vi "RightDrive.vi"(10 "Effort":dbl=-0.007874015748031496) -> ()   [LabVIEW 2018]
uses:
  <vilib>/Rock Robotics/WPI/ThirdParty/Phoenix-LabVIEW/Motor Controller/Controls/CTRE_Phoenix_MotorControl_ControlMode.ctl
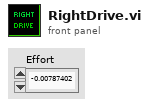
[diagram p1: front panel]
types:
  T1 = typedef "CTRE_Phoenix_MotorControl_ControlMode.ctl" = u16
  T2 = typedef "WPI_MotorControlDeviceRef.ctl" = cluster{"DeviceStatus":errorcluster, "Type":T3, "PWM":cluster{"PWM Channel":T4, "DeadBand":T5}, "CAN":cluster{"Device Number":u8, "SetOutput VI Ref":variant, "GetOutput VI Ref":variant, "Enable VI Ref":variant, "Disable VI Ref":variant, "Data":variant}, "Invert":bool, "DIO PWM":cluster{"PWM \"Enable\" Channel":T4, "DIOChannel":T6, "PWM Rate":dbl}}
  T3 = typedef "WPI_MotorControlType.ctl" = enum16{"PWM", "CAN", "DIO PWM"}
  T4 = typedef "FPGA_DIOPWMChannel.ctl" = enum8{"PWM 0", "PWM 1", "PWM 2", "PWM 3", "PWM 4", "PWM 5", "PWM 6", "PWM 7", "PWM 8", "PWM 9", "PWM MXP 0", "PWM MXP 1", "PWM MXP 2", "PWM MXP 3", "PWM MXP 4", "PWM MXP 5", "PWM MXP 6", "PWM MXP 7", "PWM MXP 8", "PWM MXP 9", "Invalid"}
  T5 = typedef "WPI_PWMDeadband.ctl" = cluster{"Name":string, "maxPositivePwm":i32, "minPositivePwm":i32, "centerPwm":i32, "maxNegativePwm":i32, "minNegativePwm":i32, "angularRange":u16}
  T6 = typedef "FPGA_DIOChannel.ctl" = enum8{"DIO 0", "DIO 1", "DIO 2", "DIO 3", "DIO 4", "DIO 5", "DIO 6", "DIO 7", "DIO 8", "DIO 9", "DIO MXP 0", "DIO MXP 1", "DIO MXP 2", "DIO MXP 3", "DIO MXP 4", "DIO MXP 5", "DIO MXP 6", "DIO MXP 7", "DIO MXP 8", "DIO MXP 9", "DIO MXP 10", "DIO MXP 11", "DIO MXP 12", "DIO MXP 13", "DIO MXP 14", "DIO MXP 15", "SPI Port CS1", "SPI Port CS2", "SPI Port CS3", "SPI Port MISO", "SPI Port MOSI", "Invalid"}
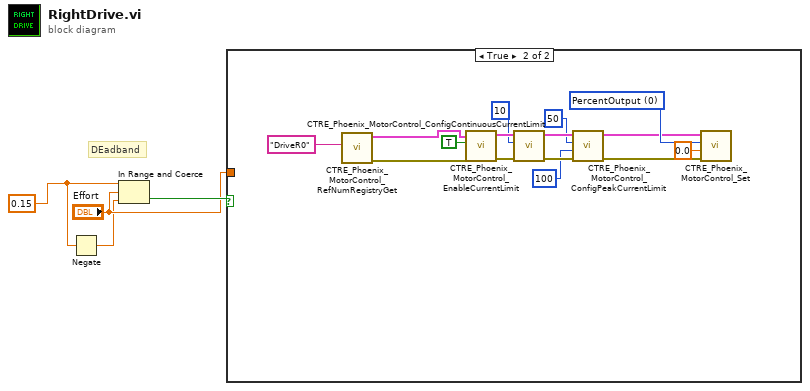
[diagram p0: block diagram]
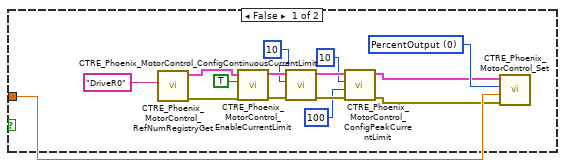
[diagram p2: hidden frame]
diagram:
  w1 = 0.15 ("upper limit")
  # "DEadband"
  n1 = Negate(x=w1) -> (-x=w2:dbl)
  n2 = In Range and Coerce(upper limit=w1, x="Effort", lower limit=w2) -> (In Range?=w4:bool)  [unwired: 1 out]
  n3 = case shown="True" w4 {
    tunnel: "Effort" -> [w17 _]
    frame False {
      w18 = T1 0 items=["PercentOutput"=0, "Position"=1, "Velocity"=2, "Current"=3, "Follower"=5, "MotionProfile"=6, "MotionMagic"=7, "MotionMagicArc"=8, "MotionProfileArc"=10, "Disabled"=15] ("Control Mode")
      n4 = call <vilib>:"CTRE_Phoenix_MotorControl_RefNumRegistryGet.vi"("refnum name"="DriveR0") -> ("error out"=w7:errorcluster, "PhoenixMotorControlDevRef"=w6:T2)  [unwired: 9 in]
      n5 = call <vilib>:"CTRE_Phoenix_MotorControl_EnableCurrentLimit.vi"("error in (no error)"=w7, "Enable Current Limit?"=TRUE, "PhoenixMotorControlDevRef"=w6) -> ("error out"=w15:errorcluster, "PhoenixMotorControlDevRef"=w14:T2)  [unwired: 7 in]
      n6 = call <vilib>:"CTRE_Phoenix_MotorControl_ConfigContinuousCurrentLimit.vi"("error in (no error)"=w15, "Continuous Current Limit (Amps)"=10, "PhoenixMotorControlDevRef"=w14) -> ("error out"=w12:errorcluster, "PhoenixMotorControlDevRef"=w13:T2)  [unwired: 7 in]
      n7 = call <vilib>:"CTRE_Phoenix_MotorControl_ConfigPeakCurrentLimit.vi"("error in (no error)"=w12, "Peak Current Maximum Duration (ms)"=100, "Peak Current (Amps)"=10, "PhoenixMotorControlDevRef"=w13) -> ("error out"=w9:errorcluster, "PhoenixMotorControlDevRef"=w8:T2)  [unwired: 6 in]
      n8 = call <vilib>:"CTRE_Phoenix_MotorControl_Set.vi"("error in (no error)"=w9, "Output"=w17, "Control Mode"=w18, "PhoenixMotorControlDevRef"=w8) -> ()  [unwired: 6 in, 2 out]
    }
    frame True {
      w33 = T1 0 items=["PercentOutput"=0, "Position"=1, "Velocity"=2, "Current"=3, "Follower"=5, "MotionProfile"=6, "MotionMagic"=7, "MotionMagicArc"=8, "MotionProfileArc"=10, "Disabled"=15] ("Control Mode")
      n9 = call <vilib>:"CTRE_Phoenix_MotorControl_RefNumRegistryGet.vi"("refnum name"="DriveR0") -> ("error out"=w23:errorcluster, "PhoenixMotorControlDevRef"=w22:T2)  [unwired: 9 in]
      n10 = call <vilib>:"CTRE_Phoenix_MotorControl_EnableCurrentLimit.vi"("error in (no error)"=w23, "Enable Current Limit?"=TRUE, "PhoenixMotorControlDevRef"=w22) -> ("error out"=w30:errorcluster, "PhoenixMotorControlDevRef"=w29:T2)  [unwired: 7 in]
      n11 = call <vilib>:"CTRE_Phoenix_MotorControl_ConfigContinuousCurrentLimit.vi"("error in (no error)"=w30, "Continuous Current Limit (Amps)"=10, "PhoenixMotorControlDevRef"=w29) -> ("error out"=w26:errorcluster, "PhoenixMotorControlDevRef"=w27:T2)  [unwired: 7 in]
      n12 = call <vilib>:"CTRE_Phoenix_MotorControl_ConfigPeakCurrentLimit.vi"("error in (no error)"=w26, "Peak Current Maximum Duration (ms)"=100, "Peak Current (Amps)"=50, "PhoenixMotorControlDevRef"=w27) -> ("error out"=w20:errorcluster, "PhoenixMotorControlDevRef"=w21:T2)  [unwired: 6 in]
      n13 = call <vilib>:"CTRE_Phoenix_MotorControl_Set.vi"("error in (no error)"=w20, "Output"=0.0, "Control Mode"=w33, "PhoenixMotorControlDevRef"=w21) -> ()  [unwired: 6 in, 2 out]
    }
  }
